vi "UNIX to Timestamp.vi"(1 "Seconds":i32) -> (0 "Timestamp String":string)   [LabVIEW 2009]
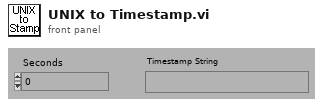
[diagram p1: front panel]
types:
  T1 = cluster{"second":i32, "minute":i32, "hour":i32, "day of month":i32, "month":i32, "year":i32, "day of week":i32, "day of year":i32, "is DST":i32}
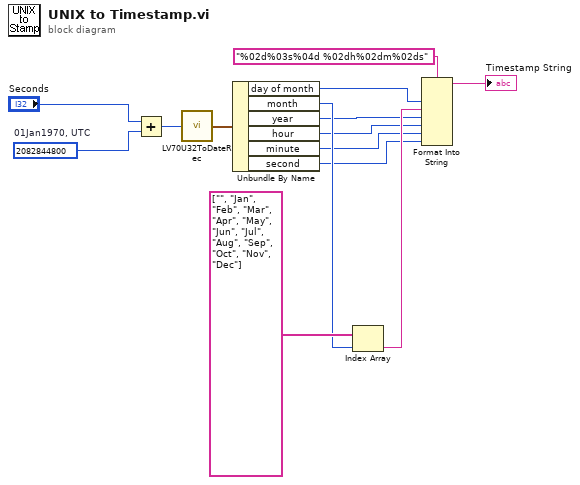
[diagram p0: block diagram]
diagram:
  w2 = 2082844800  # 01Jan1970, UTC
  n1 = Add(x="Seconds", y=w2) -> (x+y=w3:i32)
  n2 = call <vilib>:"LV70U32ToDateRec.vi"("Time"=w3) -> ("date time rec"=w14:T1)
  n3 = Unbundle By Name(w14) -> ("day of month"=w10:i32, "month"=w11:i32, "year"=w8:i32, "hour"=w7:i32, "minute"=w6:i32, "second"=w5:i32)
  n4 = Index Array(array=string[] ["", "Jan", "Feb", "Mar", "Apr", "May", "Jun", "Jul", "Aug", "Sep", "Oct", "Nov", "Dec"], index=w11) -> (element=w9:string)
  n5 = Format Into String(format string="%02d%03s%04d %02dh%02dm%02ds", w10, w9, w8, w7, w6, w5) -> (resulting string=→"Timestamp String":string)  [unwired: 2 in, 1 out]
